vi "enableLaser.vi"(8 "error in (no error)":errorcluster, 11 "Monochromator in":refnum<class "Monochromator.lvclass">) -> (0 "error out":errorcluster, 1 "ID":i32, 2 "results-JSON string":string, 3 "Monochromator out":refnum<class "Monochromator.lvclass">)   [LabVIEW 2023, in "Monochromator.lvclass"]
uses:
  Monochromator.lvclass
  7fe8abea-6ecd-46de-aa11-ce8637911b6a.vi
  35d46a5a-fd7c-4445-96f4-e877dae8f93b.vi
  <vilib>/JDP Science/JSONtext/Variant to JSON Text.vi
  <vilib>/JDP Science/JSONtext/Set Item.vi
  <vilib>/JDP Science/JSONtext/LVClass Serializer/JSONtext LVClass Serializer.lvclass
  Monochromator.lvclass/Monochromator.ctl
  GenericDevice/GenericDevice.lvclass
  <vilib>/IlluminatedG/lv-web-crypto/lv-json/JSON/JSON.lvlib
panel:
  # "Connector Pane"
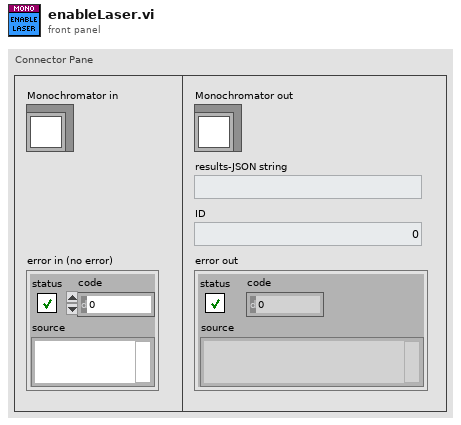
[diagram p1: front panel]
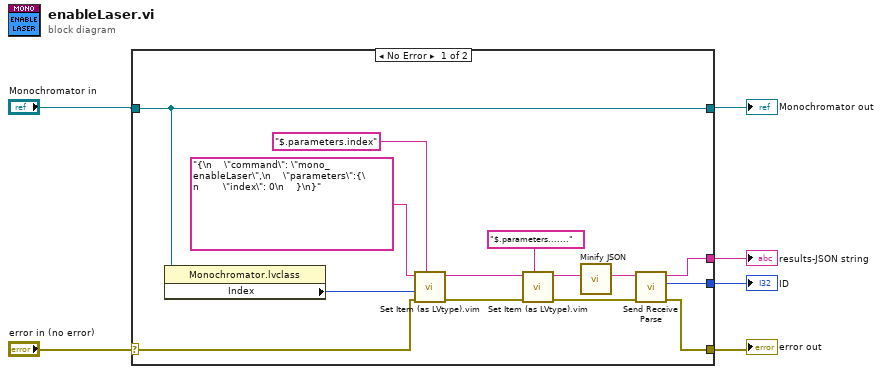
[diagram p0: block diagram]
diagram:
  n1 = case shown="No Error" "error in (no error)" {
    selector: "error in (no error)" -> [w16 w22]
    tunnel: [w13 w22] -> w3
    tunnel: [w18 w21] -> w5
    tunnel: "Monochromator in" -> [w18 w21]
    tunnel: [w15 _] -> w1
    tunnel: [w14 _] -> w2
    frame No Error {
      n2 = property class="Monochromator.lvclass"(reference=w18) -> ("Index"=w17:i32)  [unwired: 1 in, 2 out]
      n3 = call "Set Item (as LVtype).vim"("$Path or Item Name"="$.parameters.index", "error in (no error)"=w16, "Anything"=w17, "JSON"="{\n    \"command\": \"mono_enableLaser\",\n    \"parameters\":{\n        \"index\": 0\n    }\n}") -> ("error out"=w10:errorcluster, "<JSON>"=w8:string)  [unwired: 4 in, 1 out]
      n4 = call "Set Item (as LVtype).vim"("$Path or Item Name"="$.parameters.......", "error in (no error)"=w10, "JSON"=w8) -> ("error out"=w9:errorcluster, "<JSON>"=w7:string)  [unwired: 5 in, 1 out]
      n5 = call <vilib>:"Minify JSON.vi"("JSON String"=w7) -> ("Minified JSON"=w12:string)  [unwired: 10 in]
      n6 = call "Send Receive Parse.vi"("error in"=w9, "<JSON>"=w12) -> ("error out"=w13:errorcluster, "ID"=w14:i32, "results-JSON string"=w15:string)  [unwired: 7 in]
    }
    frame Error {
    }
  }
  "error out" <- w3
  "Monochromator out" <- w5
  "ID" <- w2
  "results-JSON string" <- w1
